vi "ExtraTreeClassifier.vi"(8 "error in":errorcluster) -> (0 "error out":errorcluster, 3 "out":refnum<class "ExtraTreeClassifier.lvclass">)   [LabVIEW 2020]
doc: "An extremely randomized tree classifier.\n\n Extra-trees differ from classic decision trees in the way they are built.\n When looking for the best split to separate the samples of a node into two\n groups, random splits are drawn for each of the `max_features` randomly\n selected features and the best split among those is chosen. When\n `max_features` is set 1, this amounts to building a totally random\n decision tree.\n\n Warning: Extra-trees should only be used within ensemble methods.\n\n Read more in the :ref:`User Guide <tree>`.\n\n Parameters\n ----------\n criterion : {\"gini\", \"entropy\"}, default=\"gini\"\n The function to measure the quality of a split. Supported criteria are\n \"gini\" for the Gini impurity and \"entropy\" for the information gain.\n\n splitter : {\"random\", \"best\"}, default=\"random\"\n The strategy used to choose the split at each node. Supported\n strategies are \"best\" to choose the best split and \"random\" to choose\n the best random split.\n\n max_depth : int, default=None\n The maximum depth of the tree. If None, then nodes are expanded until\n all leaves are pure or until all leaves contain less than\n min_samples_split samples.\n\n min_samples_split : int or float, default=2\n The minimum number of samples required to split an internal node:\n\n - If int, then consider `min_samples_split` as the minimum number.\n - If float, then `min_samples_split` is a fraction and\n `ceil(min_samples_split * n_samples)` are the minimum\n number of samples for each split.\n\n .. versionchanged:: 0.18\n Added float values for fractions.\n\n min_samples_leaf : int or float, default=1\n The minimum number of samples required to be at a leaf node.\n A split point at any depth will only be considered if it leaves at\n least ``min_samples_leaf`` training samples in each of the left and\n right branches. This may have the effect of smoothing the model,\n especially in regression.\n\n - If int, then consider `min_samples_leaf` as the minimum number.\n - If float, then `min_samples_leaf` is a fraction and\n `ceil(min_samples_leaf * n_samples)` are the minimum\n number of samples for each node.\n\n .. versionchanged:: 0.18\n Added float values for fractions.\n\n min_weight_fraction_leaf : float, default=0.0\n The minimum weighted fraction of the sum total of weights (of all\n the input samples) required to be at a leaf node. Samples have\n equal weight when sample_weight is not provided.\n\n max_features : int, float, {\"auto\", \"sqrt\", \"log2\"} or None, default=\"auto\"\n The number of features to consider when looking for the best split:\n\n - If int, then consider `max_features` features at each split.\n - If float, then `max_features` is a fraction and\n `int(max_features * n_features)` features are considered at each\n split.\n - If \"auto\", then `max_features=sqrt(n_features)`.\n - If \"sqrt\", then `max_features=sqrt(n_features)`.\n - If \"log2\", then `max_features=log2(n_features)`.\n - If None, then `max_features=n_features`.\n\n Note: the search for a split does not stop until at least one\n valid partition of the node samples is found, even if it requires to\n effectively inspect more than ``max_features`` features.\n\n random_state : int, RandomState instance or None, default=None\n Used to pick randomly the `max_features` used at each split.\n See :term:`Glossary <random_state>` for details.\n\n max_leaf_nodes : int, default=None\n Grow a tree with ``max_leaf_nodes`` in best-first fashion.\n Best nodes are defined as relative reduction in impurity.\n If None then unlimited number of leaf nodes.\n\n min_impurity_decrease : float, default=0.0\n A node will be split if this split induces a decrease of the impurity\n greater than or equal to this value.\n\n The weighted impurity decrease equation is the following::\n\n N_t / N * (impurity - N_t_R / N_t * right_impurity\n - N_t_L / N_t * left_impurity)\n\n where ``N`` is the total number of samples, ``N_t`` is the number of\n samples at the current node, ``N_t_L`` is the number of samples in the\n left child, and ``N_t_R`` is the number of samples in the right child.\n\n ``N``, ``N_t``, ``N_t_R`` and ``N_t_L`` all refer to the weighted sum,\n if ``sample_weight`` is passed.\n\n .. versionadded:: 0.19\n\n min_impurity_split : float, default=None\n Threshold for early stopping in tree growth. A node will split\n if its impurity is above the threshold, otherwise it is a leaf.\n\n .. deprecated:: 0.19\n ``min_impurity_split`` has been deprecated in favor of\n ``min_impurity_decrease`` in 0.19. The default value of\n ``min_impurity_split`` has changed from 1e-7 to 0 in 0.23 and it\n will be removed in 1.0 (renaming of 0.25).\n Use ``min_impurity_decrease`` instead.\n\n class_weight : dict, list of dict or \"balanced\", default=None\n Weights associated with classes in the form ``{class_label: weight}``.\n If None, all classes are supposed to have weight one. For\n multi-output problems, a list of dicts can be provided in the same\n order as the columns of y.\n\n Note that for multioutput (including multilabel) weights should be\n defined for each class of every column in its own dict. For example,\n for four-class multilabel classification weights should be\n [{0: 1, 1: 1}, {0: 1, 1: 5}, {0: 1, 1: 1}, {0: 1, 1: 1}] instead of\n [{1:1}, {2:5}, {3:1}, {4:1}].\n\n The \"balanced\" mode uses the values of y to automatically adjust\n weights inversely proportional to class frequencies in the input data\n as ``n_samples / (n_classes * np.bincount(y))``\n\n For multi-output, the weights of each column of y will be multiplied.\n\n Note that these weights will be multiplied with sample_weight (passed\n through the fit method) if sample_weight is specified.\n\n ccp_alpha : non-negative float, default=0.0\n Complexity parameter used for Minimal Cost-Complexity Pruning. The\n subtree with the largest cost complexity that is smaller than\n ``ccp_alpha`` will be chosen. By default, no pruning is performed. See\n :ref:`minimal_cost_complexity_pruning` for details.\n\n .. versionadded:: 0.22\n\n Attributes\n ----------\n classes_ : ndarray of shape (n_classes,) or list of ndarray\n The classes labels (single output problem),\n or a list of arrays of class labels (multi-output problem).\n\n max_features_ : int\n The inferred value of max_features.\n\n n_classes_ : int or list of int\n The number of classes (for single output problems),\n or a list containing the number of classes for each\n output (for multi-output problems).\n\n feature_importances_ : ndarray of shape (n_features,)\n The impurity-based feature importances.\n The higher, the more important the feature.\n The importance of a feature is computed as the (normalized)\n total reduction of the criterion brought by that feature. It is also\n known as the Gini importance.\n\n Warning: impurity-based feature importances can be misleading for\n high cardinality features (many unique values). See\n :func:`sklearn.inspection.permutation_importance` as an alternative.\n\n n_features_ : int\n The number of features when ``fit`` is performed.\n\n n_outputs_ : int\n The number of outputs when ``fit`` is performed.\n\n tree_ : Tree instance\n The underlying Tree object. Please refer to\n ``help(sklearn.tree._tree.Tree)`` for attributes of Tree object and\n :ref:`sphx_glr_auto_examples_tree_plot_unveil_tree_structure.py`\n for basic usage of these attributes.\n\n See Also\n --------\n ExtraTreeRegressor : An extremely randomized tree regressor.\n sklearn.ensemble.ExtraTreesClassifier : An extra-trees classifier.\n sklearn.ensemble.ExtraTreesRegressor : An extra-trees regressor.\n\n Notes\n -----\n The default values for the parameters controlling the size of the trees\n (e.g. ``max_depth``, ``min_samples_leaf``, etc.) lead to fully grown and\n unpruned trees which can potentially be very large on some data sets. To\n reduce memory consumption, the complexity and size of the trees should be\n controlled by setting those parameter values.\n\n References\n ----------\n\n .. [1] P. Geurts, D. Ernst., and L. Wehenkel, \"Extremely randomized trees\",\n Machine Learning, 63(1), 3-42, 2006.\n\n \nAvailable methods:\nApply\nCost Complexity Pruning Path\nDecision Path\nFit\nGet Depth\nGet N Leaves\nPredict\nScore\nGet Attributes\nGet Params\nSet Params"
uses:
  ExtraTreeClassifier.lvclass
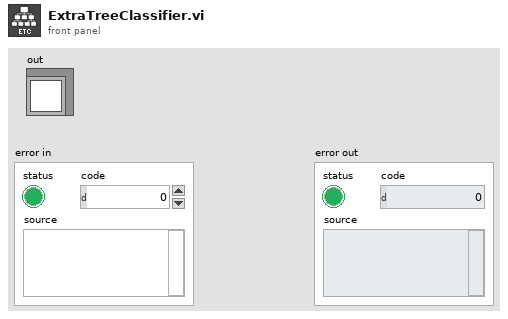
[diagram p1: front panel]
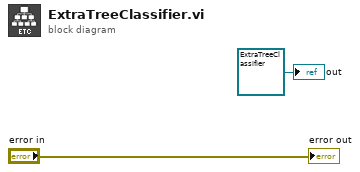
[diagram p0: block diagram]
diagram:
  "out" <- refnum<class "ExtraTreeClassifier.lvclass"> refnum ("model")
  "error out" <- "error in"
